vi "linear interp iiii- complex - z-omega - divide.vi"(0 "z":cdb[](array[numeric]), 1 "number of segments":i32=3, 5 "omega":dbl[](array[numeric]), 11 "center":i32=-1) -> (2 "directed sigma":cdb, 3 "directed sigma - abs":dbl, 4 "z out":cdb[](array[numeric]), 6 "omega out":dbl[](array[numeric]), 8 "left":cdb, 10 "center":cdb, 12 "intercept":cdb, 13 "slope":cdb, 14 "phase rotation":dbl, 15 "right":cdb)   [LabVIEW 2017]
uses:
  <vilib>/Analysis/baseanly.llb/A x B.vi
  <vilib>/Analysis/baseanly.llb/Complex A x B.vi
  Q -- check range -- i -- real.vi
  Q - not nan -- integer.vi
  Q - not nan -- real.vi
  <vilib>/Analysis/baseanly.llb/Inverse Matrix.vi
  <vilib>/Analysis/baseanly.llb/Real Inverse Matrix.vi
  <vilib>/Analysis/Matrix/Numeric/Conversions/Array To Matrix.vi
  <vilib>/Analysis/Matrix/Numeric/Conversions/Array To Matrix - RA2.vi
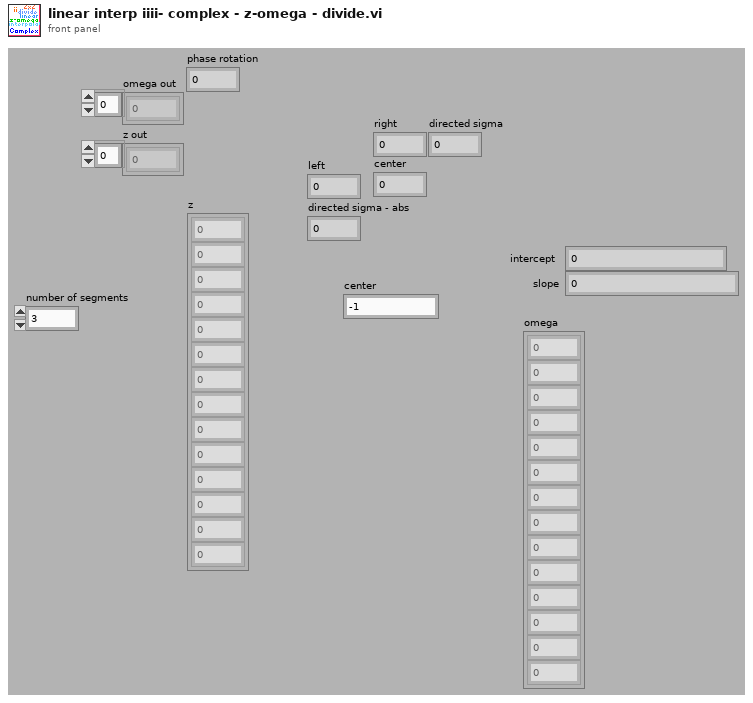
[diagram p1: front panel]
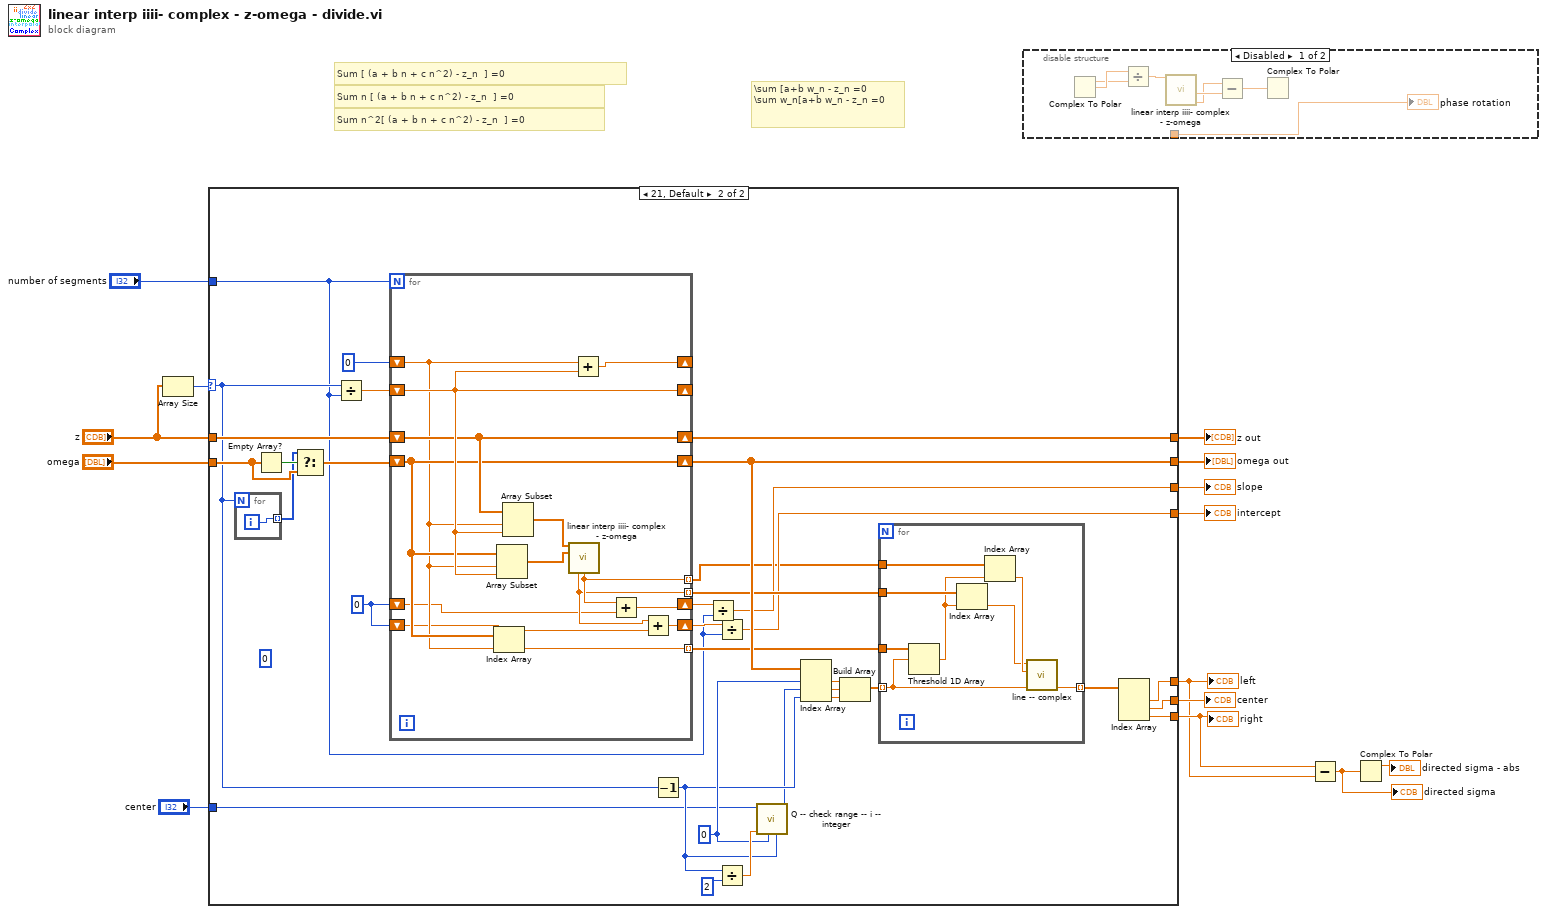
[diagram p0: block diagram]
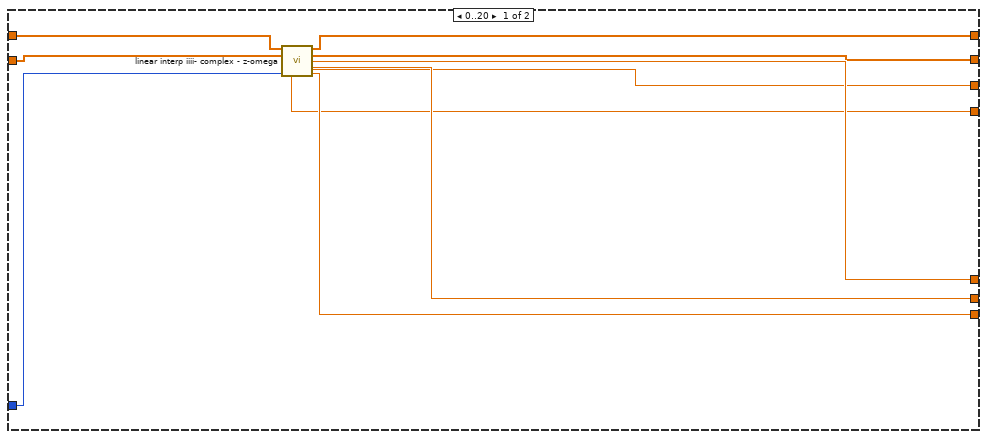
[diagram p3: hidden frame]
diagram:
  # "\\sum [a+b w_n - z_n =0 \n\\sum w_n[a+b w_n - z_n =0"
  # "Sum n^2[ (a + b n + c n^2) - z_n  ] =0"
  # "Sum n [ (a + b n + c n^2) - z_n  ] =0"
  # "Sum [ (a + b n + c n^2) - z_n  ] =0"
  n1 = Array Size(array="z") -> (size(s)=w11:i32)
  n2 = case shown="21, Default" w11 {
    selector: w11 -> [_ w47]
    tunnel: "z" -> [w24 w54]
    tunnel: "omega" -> [w23 w56]
    tunnel: [w17 w46] -> w9
    tunnel: [w18 w50] -> w8
    tunnel: "center" -> [w22 w43]
    tunnel: [w20 w35] -> w4
    tunnel: [w19 w34] -> w6
    tunnel: [w21 w33] -> w5
    tunnel: [w16 w28] -> w3
    tunnel: [w15 w27] -> w2
    tunnel: "number of segments" -> [_ w26]
    frame 0..20 {
      n3 = call "linear interp iiii- complex - z-omega.vi"("z"=w24, "omega"=w23, "center"=w22) -> ("z out"=w18:cdb[], "omega out"=w17:dbl[], "left"=w20:cdb, "center"=w19:cdb, "intercept"=w15:cdb, "slope"=w16:cdb, "right"=w21:cdb)  [unwired: 4 in, 2 out]
    }
    frame 21, Default {
      (unwired) 0 ("y")
      w31 = 0 ("y")
      w45 = 0 ("n")
      n4 = for {
        N: w47 -> [_]
        tunnel: [w80] -> w55 mode=indexing
        i -> [w80]
      }
      n5 = Empty Array?(array=w56) -> (empty?=w57:bool)
      n6 = Select(t=w55, s=w57, f=w56) -> (s? t:f=w53:dbl[])
      n7 = Divide(x=w47, y=w26) -> (x/y=w51:dbl)
      n8 = for {
        N: w26 -> [_]
        tunnel: [w70] -> w36 mode=indexing
        tunnel: [w71] -> w25 mode=indexing
        shift-right: [w79] -> _
        shift-left: 0 ("y") -> [w73]
        shift-right: [w75] -> w50
        shift-left: w54 -> [w75]
        shift-right: [w74] -> w46
        shift-left: w53 -> [w74]
        shift-right: [w78] -> _
        shift-left: w51 -> [w78]
        tunnel: [w72] -> w37 mode=indexing
        shift-right: [w69] -> w30
        shift-left: w31 -> [w66]
        shift-right: [w68] -> w29
        shift-left: w31 -> [w67]
        n9 = Index Array(array=w74, index=w73) -> (element=w72:dbl)
        n10 = Array Subset(array=w74, index=w73, length=w78) -> (w76:dbl[])
        n11 = Array Subset(array=w75, index=w73, length=w78) -> (w77:cdb[])
        n12 = call "linear interp iiii- complex - z-omega.vi"("z"=w77, "omega"=w76) -> ("intercept"=w70:cdb, "slope"=w71:cdb)  [unwired: 5 in, 7 out]
        n13 = Add(x=w73, y=w78) -> (x+y=w79:dbl)
        n14 = Add(x=w71, y=w66) -> (x+y=w69:cdb)
        n15 = Add(x=w70, y=w67) -> (x+y=w68:cdb)
      }
      n16 = Decrement(x=w47) -> (x-1=w44:i32)
      n17 = Divide(x=w30, y=w26) -> (x/y=w28:cdb)
      n18 = Divide(x=w29, y=w26) -> (x/y=w27:cdb)
      n19 = Divide(x=w44, y=2 ("n")) -> (x/y=w49:dbl)
      n20 = call "Q -- check range -- i -- integer.vi"("upper"=w44, "lower"=w45, "default"=w49, "number"=w43) -> ("number in range"=w42:i32)  [unwired: 5 in, 2 out]
      n21 = Index Array(array=w46, index #1=w45, index #2=w42, index #3=w44) -> (element #1=w41:dbl, element #2=w40:dbl, element #3=w39:dbl)
      n22 = Build Array(w41, w40, w39) -> (w38:dbl[])
      n23 = for {
        tunnel: w38 -> [w58] mode=indexing
        tunnel: w37 -> [w65]
        tunnel: w25 -> [w64]
        tunnel: w36 -> [w63]
        tunnel: [w61] -> w32 mode=indexing
        n24 = Threshold 1D Array(2:w58, 3:w65) -> (0:w62:dbl)  [unwired: 1 in]
        n25 = Index Array(array=w63, index=w62) -> (element=w59:cdb)
        n26 = Index Array(array=w64, index=w62) -> (element=w60:cdb)
        n27 = call "line -- complex.vi"("n"=w58, "slope"=w60, "intercept"=w59) -> ("value"=w61:cdb)  [unwired: 7 in, 1 out]
      }
      n28 = Index Array(array=w32) -> (element #1=w35:cdb, element #2=w34:cdb, element #3=w33:cdb)  [unwired: 3 in]
    }
  }
  "slope" <- w3
  "intercept" <- w2
  "left" <- w4
  "right" <- w5
  "center" <- w6
  "omega out" <- w9
  "z out" <- w8
  n29 = disable-structure shown="Disabled" {
    disable-tunnel: _ -> [w88 _]
    frame Disabled {
      n30 = Complex To Polar() -> (r * e^(i*theta)=w82:cdb, r=w81:dbl)  [unwired: 1 out]
      n31 = Divide(x=w82, y=w81) -> (x/y=w83:dbl)
      n32 = call "linear interp iiii- complex - z-omega.vi"("z"=w83) -> ("left"=w86:cdb, "right"=w85:cdb)  [unwired: 6 in, 7 out]
      n33 = Subtract(x=w85, y=w86) -> (x-y=w84:cdb)
      n34 = Complex To Polar(r * e^(i*theta)=w84) -> (r=w87:dbl)  [unwired: 1 out]
      "phase rotation" <- w88
    }
    frame Enabled {
    }
  }
  n35 = Subtract(x=w5, y=w4) -> (x-y=w13:cdb)
  "directed sigma" <- w13
  n36 = Complex To Polar(r * e^(i*theta)=w13) -> (r=→"directed sigma - abs":dbl)  [unwired: 1 out]
